vi "AutoScale.vi"(3 "Channel 1 Enable":bool, 6 "Channel 0 Enable":bool) -> (0 "Scale\n  Volts/Div 1":dbl(knob)=0.5 scale=0.01..20.0, 1 "Time/Div":dbl(knob)=5e-06 scale=5e-06..0.2, 2 "Scale\n  Volts/Div 0":dbl(knob)=0.5 scale=0.01..20.0)   [LabVIEW 2012]
uses:
  GlobalVariable.vi
panel:
  out "Timebase":dbl[](array[numeric])=[5e-06, 1e-05, 2e-05, 5e-05, 0.0001, 0.0002, 0.0005, 0.001, 0.002, 0.005, 0.01, 0.02, 0.05, 0.1, 0.2]
  out "Volts":dbl[](array[numeric])=[0.01, 0.02, 0.05, 0.1, 0.2, 0.5, 1.0, 2.0, 5.0, 10.0, 20.0]
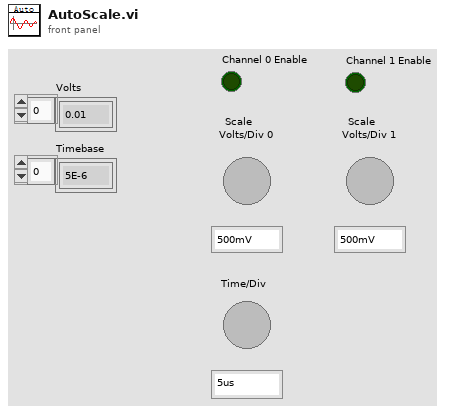
[diagram p1: front panel]
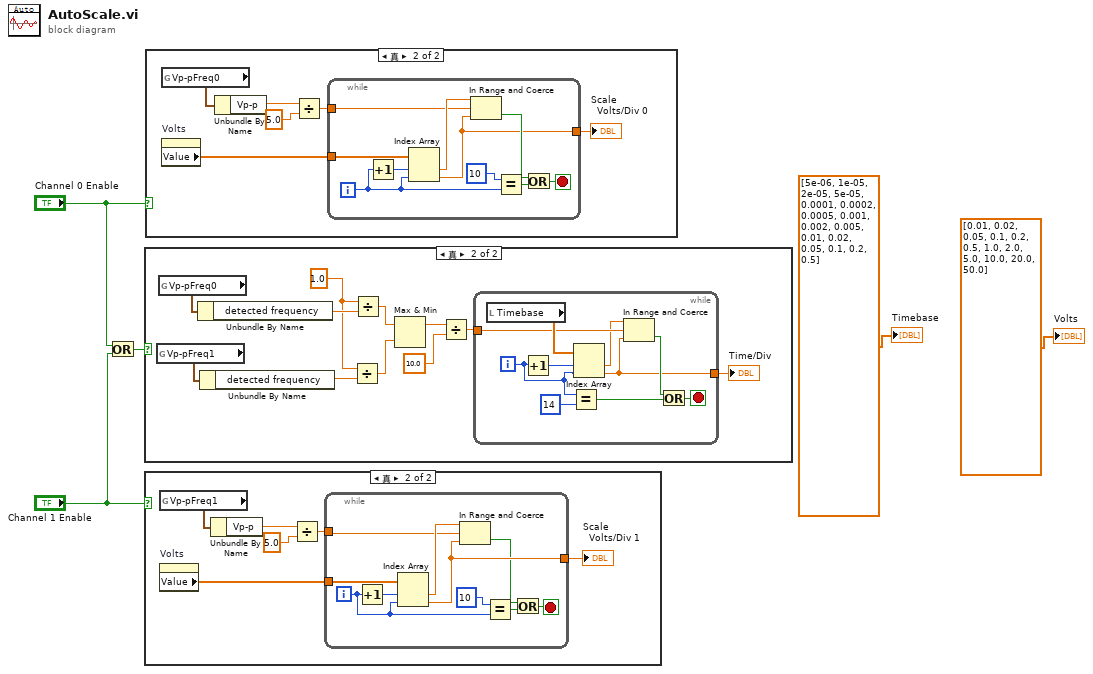
[diagram p0: block diagram]
diagram:
  n1 = Or(x="Channel 0 Enable", y="Channel 1 Enable") -> (x .or. y?=w3:bool)
  n2 = case shown="真" w3 {
    frame False {
    }
    frame True {
      w14 = 1.0 ("x")
      n3 = global read "GlobalVariable.vi" "Vp-pFreq1"() -> (w9:cluster{"Vp-p":dbl, "detected frequency":dbl})
      n4 = global read "GlobalVariable.vi" "Vp-pFreq0"() -> (w10:cluster{"Vp-p":dbl, "detected frequency":dbl})
      n5 = Unbundle By Name(w10) -> ("detected frequency"=w16:dbl)
      n6 = Unbundle By Name(w9) -> ("detected frequency"=w15:dbl)
      n7 = Divide(x=w14, y=w15) -> (x/y=w12:dbl)
      n8 = Divide(x=w14, y=w16) -> (x/y=w13:dbl)
      n9 = Max & Min(x=w13, y=w12) -> (max(x,y)=w8:dbl)  [unwired: 1 out]
      n10 = Divide(x=w8, y=10.0) -> (x/y=w6:dbl)
      n11 = while {
        tunnel: w6 -> [w25]
        tunnel: [w17] -> w11
        i -> [w19]
        stop <- w21 stop-if-true
        n12 = local read "Timebase"() -> (w26:dbl[])
        n13 = Increment(x=w19) -> (x+1=w20:i32)
        n14 = Equal?(x=w19, y=14) -> (x = y?=w23:bool)
        n15 = Index Array(array=w26, index #1=w20, index #2=w19) -> (element #1=w18:dbl, element #2=w17:dbl)
        n16 = In Range and Coerce(upper limit=w18, x=w25, lower limit=w17) -> (In Range?=w22:bool)  [unwired: 1 out]
        n17 = Or(x=w22, y=w23) -> (x .or. y?=w21:bool)
      }
      "Time/Div" <- w11
    }
  }
  n18 = case shown="真" "Channel 1 Enable" {
    frame False {
    }
    frame True {
      n19 = global read "GlobalVariable.vi" "Vp-pFreq1"() -> (w28:cluster{"Vp-p":dbl, "detected frequency":dbl})
      n20 = property on="Volts" class="Arr (严格)"() -> ("Value"=w29:dbl[])  [unwired: 2 in, 2 out]
      n21 = Unbundle By Name(w28) -> ("Vp-p"=w31:dbl)
      n22 = Divide(x=w31, y=5.0) -> (x/y=w30:dbl)
      n23 = while {
        tunnel: w30 -> [w38]
        tunnel: w29 -> [w41]
        tunnel: [w37] -> w27
        i -> [w34]
        stop <- w42 stop-if-true
        n24 = Increment(x=w34) -> (x+1=w39:i32)
        n25 = Index Array(array=w41, index #1=w39, index #2=w34) -> (element #1=w40:dbl, element #2=w37:dbl)
        n26 = In Range and Coerce(upper limit=w40, x=w38, lower limit=w37) -> (In Range?=w36:bool)  [unwired: 1 out]
        n27 = Equal?(x=10, y=w34) -> (x = y?=w35:bool)
        n28 = Or(x=w36, y=w35) -> (x .or. y?=w42:bool)
      }
      "Scale\n  Volts/Div 1" <- w27
    }
  }
  n29 = case shown="真" "Channel 0 Enable" {
    frame False {
    }
    frame True {
      n30 = global read "GlobalVariable.vi" "Vp-pFreq0"() -> (w44:cluster{"Vp-p":dbl, "detected frequency":dbl})
      n31 = property on="Volts" class="Arr (严格)"() -> ("Value"=w45:dbl[])  [unwired: 2 in, 2 out]
      n32 = Unbundle By Name(w44) -> ("Vp-p"=w48:dbl)
      n33 = Divide(x=w48, y=5.0) -> (x/y=w46:dbl)
      n34 = while {
        tunnel: w46 -> [w53]
        tunnel: [w50] -> w43
        tunnel: w45 -> [w52]
        i -> [w51]
        stop <- w49 stop-if-true
        n35 = Increment(x=w51) -> (x+1=w55:i32)
        n36 = Index Array(array=w52, index #1=w55, index #2=w51) -> (element #1=w54:dbl, element #2=w50:dbl)
        n37 = In Range and Coerce(upper limit=w54, x=w53, lower limit=w50) -> (In Range?=w56:bool)  [unwired: 1 out]
        n38 = Equal?(x=10, y=w51) -> (x = y?=w57:bool)
        n39 = Or(x=w56, y=w57) -> (x .or. y?=w49:bool)
      }
      "Scale\n  Volts/Div 0" <- w43
    }
  }
  "Volts" <- dbl[] [0.01, 0.02, 0.05, 0.1, 0.2, 0.5, 1.0, 2.0, 5.0, 10.0, 20.0, 50.0]
  "Timebase" <- dbl[] [5e-06, 1e-05, 2e-05, 5e-05, 0.0001, 0.0002, 0.0005, 0.001, 0.002, 0.005, 0.01, 0.02, 0.05, 0.1, 0.2, 0.5]
